vi "Calculate Setpoint.vi"(8 "error in (no error)":errorcluster, 10 "time (sec)":dbl, 11 "Open-Loop Setpoint in":refnum<class "Open-Loop Setpoint.lvclass">) -> (0 "error out":errorcluster, 2 "setpoint":dbl, 3 "Open-Loop Setpoint out":refnum<class "Open-Loop Setpoint.lvclass">, 5 "testing?":bool)   [LabVIEW 2020, in "Open-Loop Setpoint.lvclass"]
uses:
  Open-Loop Setpoint.lvclass
  Open-Loop Setpoint.lvclass/Open-Loop Setpoint.ctl
  IA Test Parameters.lvclass
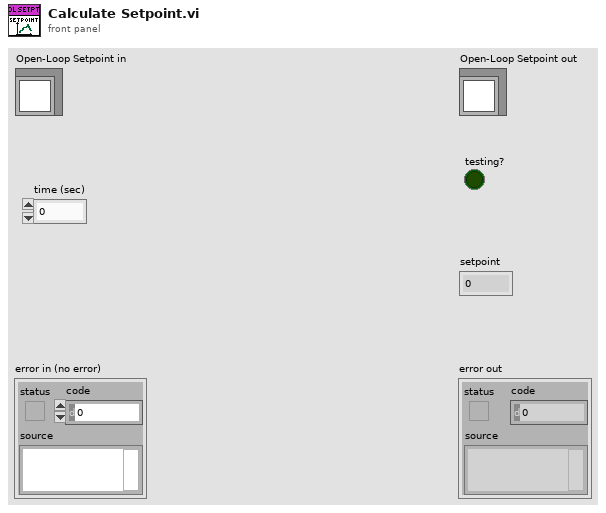
[diagram p1: front panel]
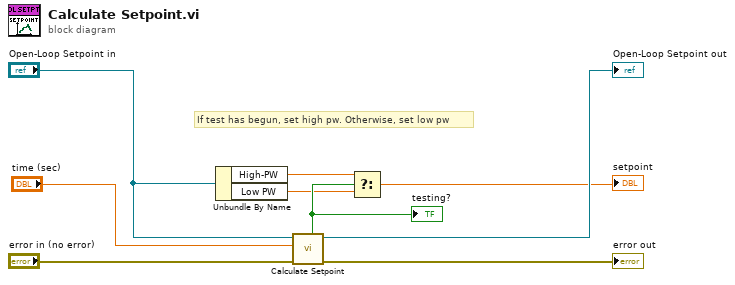
[diagram p0: block diagram]
diagram:
  # "If test has begun, set high pw. Otherwise, set low pw"
  n1 = Unbundle By Name("Open-Loop Setpoint in") -> ("High-PW"=w7:dbl, "Low PW"=w1:dbl)
  n2 = call-parent "Calculate Setpoint.vi"("error in (no error)"="error in (no error)", "time (sec)"="time (sec)", "IA Test Parameters in"="Open-Loop Setpoint in") -> ("error out"=→"error out":errorcluster, "IA Test Parameters out"=→"Open-Loop Setpoint out":refnum<class "Open-Loop Setpoint.lvclass">, "testing?"=w5:bool)  [unwired: 5 in, 1 out]
  "testing?" <- w5
  n3 = Select(t=w7, s=w5, f=w1) -> (s? t:f=→"setpoint":dbl)
